vi "Remove Chassis.vi"(0 "session in":refnum<k21>, 5 "chassis":refnum<k21>, 11 "error in (no error)":errorcluster) -> (4 "session out":refnum<k21>, 15 "error out":errorcluster)   [LabVIEW 2020, in "SLSC.lvlib"]
doc: "Removes the specified chassis from the local configuration file. Note that if the system and the SLSC chassis are on the same network subnet, then the SLSC driver will discover the chassis via mDNS and it will continue to show up in SLSC I/O controls, the Sys.Devices property, etc."
uses:
  <vilib>/SLSC/SLSC.lvlib
  nislsclvapi.dll
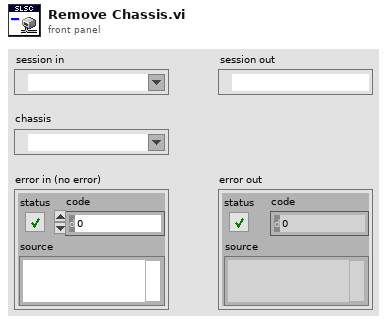
[diagram p1: front panel]
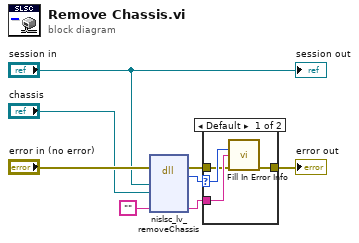
[diagram p0: block diagram]
diagram:
  n1 = dll-call lib="nislsclvapi.*" fn="nislsc_lv_removeChassis"(error in="error in (no error)", "session"="session in", "chassis"="chassis", "extendedErrorInfo"="") -> (error out=w5:errorcluster, "return type"=w4:i32, "extendedErrorInfo"=w6:string)  [unwired: 6 in, 1 out]
  n2 = case shown="Default" w4 {
    selector: w4 -> [w12 _]
    tunnel: w6 -> [w11 _]
    tunnel: w5 -> [w10 w13]
    tunnel: [w9 w13] -> w3
    frame Default {
      n3 = call <vilib>:"Fill In Error Info.vi"("status code"=w12, "extended error info"=w11, "error in"=w10) -> ("error out"=w9:errorcluster)  [unwired: 12 in]
    }
    frame 0 {
    }
  }
  "error out" <- w3
  "session out" <- "session in"
